vi "ReadPoti.vi"(11 "Potentiometers":dbl[](array[numeric])) -> (0 "LeftPotiVolt[V]":dbl, 1 "RightPotiVolt[V]":dbl, 2 "PotiPosTrans[mm]":dbl, 3 "PotiPosRot[°]":dbl)   [LabVIEW 2019]
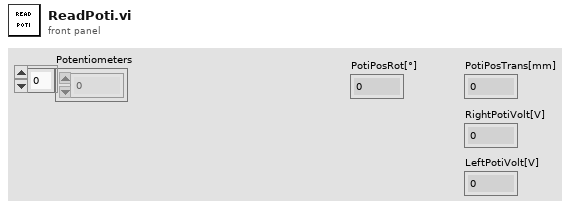
[diagram p1: front panel]
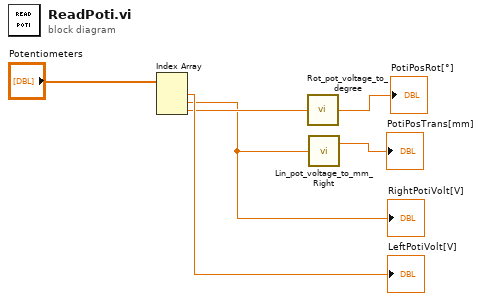
[diagram p0: block diagram]
diagram:
  n1 = Index Array(array="Potentiometers") -> (element #1=→"LeftPotiVolt[V]":dbl, element #2=w1:dbl, element #3=w3:dbl)  [unwired: 3 in]
  "RightPotiVolt[V]" <- w1
  n2 = call "Rot_pot_voltage_to_degree.vi"("RotaryPot (Voltage)"=w3) -> ("RotaryPot (degree)"=→"PotiPosRot[°]":dbl)
  n3 = call "Lin_pot_voltage_to_mm_Right.vi"("LinPot Voltage"=w1) -> ("LinPot mm (finger to finger)"=→"PotiPosTrans[mm]":dbl)  [unwired: 1 out]
